vi "Write_Results_file.vi"(0 "Experiment start time":dbl, 1 "Experiment End time":dbl, 3 "Setup filename":string) -> ()   [LabVIEW 2010]
uses:
  Controls/Post_Process.ctl
  Globals/Meas_global.vi
  Globals/Trav_pos_global.vi
  Globals/Dynamic_call_global.ph.vi
panel:
  out "x-y":u32
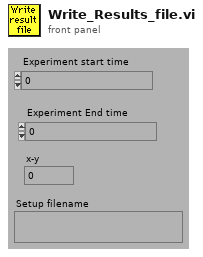
[diagram p1: front panel]
types:
  T1 = typedef "Post_Process.ctl" = enum16{"Take New Data", "Post Process Raw Data File"}
  T2 = cluster{"Name":string, "X":dbl, "Y":dbl, "Z":dbl}[]
  T3 = enum16{"Save no data", "Save data in new files", "Save data in existing files"}
  T4 = typedef "Velocity_cluster.ctl" = cluster{"Name":string, "U":dbl, "u^2":dbl, "u^3/(u^2)^(1.5)":dbl, "u^4/(u^2)^2 -3":dbl, "% u'/U":dbl, "Mean % Err":dbl, "u^4":dbl}
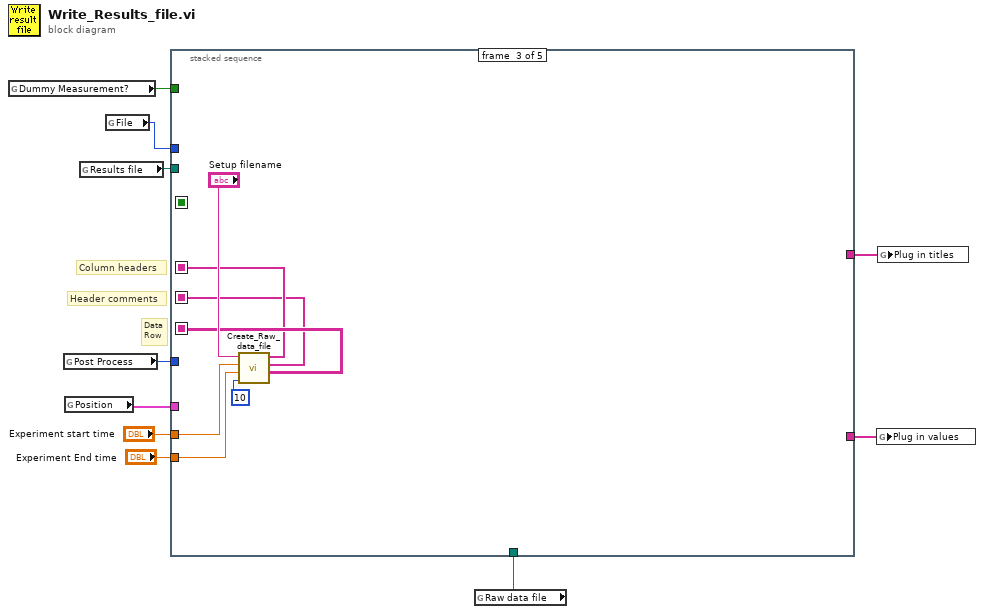
[diagram p0: block diagram]
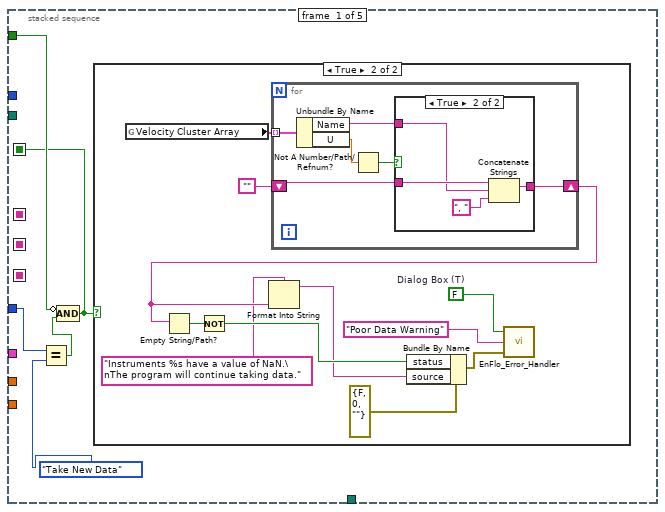
[diagram p2: hidden frame]
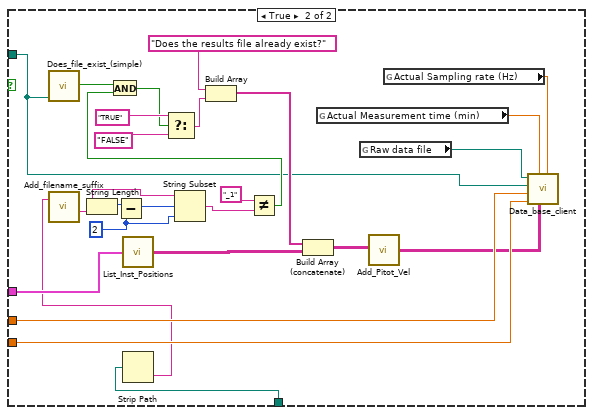
[diagram p6: hidden frame]
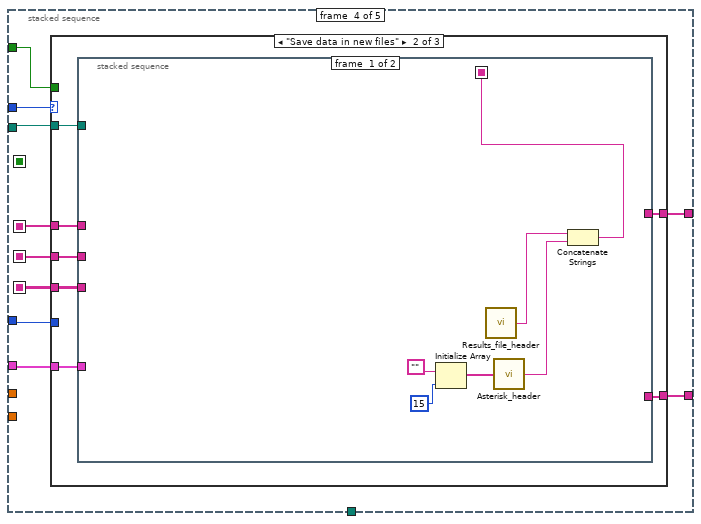
[diagram p7: hidden frame]
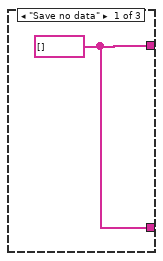
[diagram p8: hidden frame]
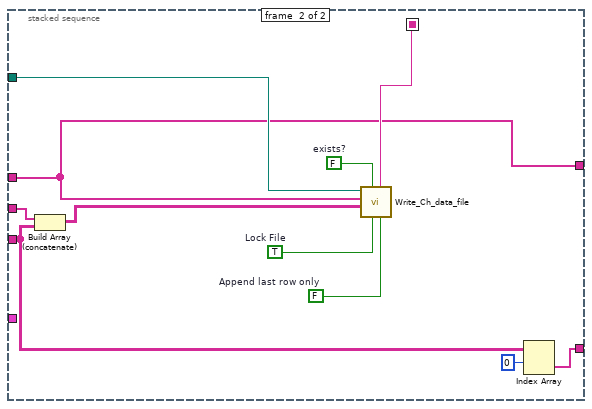
[diagram p9: hidden frame]
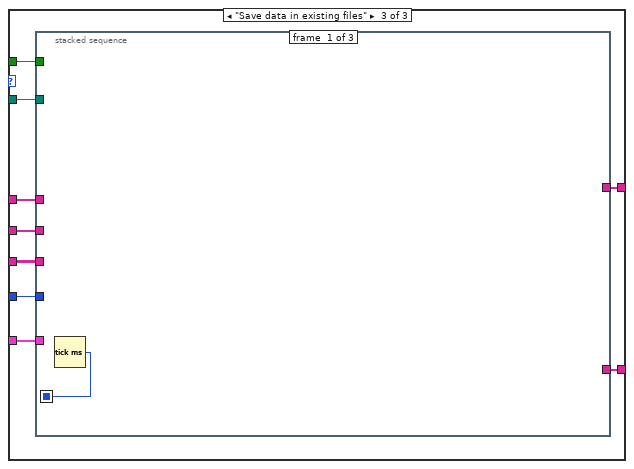
[diagram p10: hidden frame]
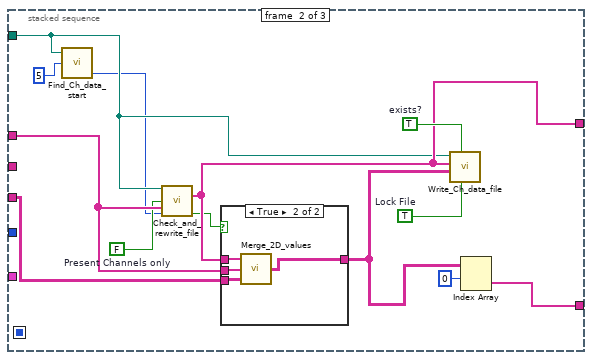
[diagram p11: hidden frame]
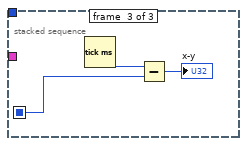
[diagram p13: hidden frame]
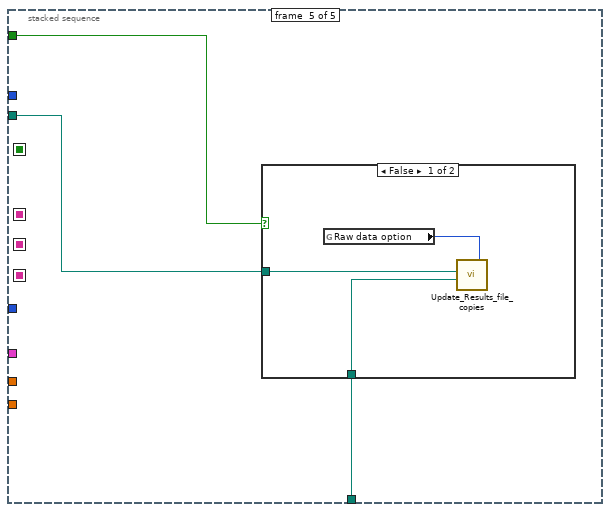
[diagram p14: hidden frame]
diagram:
  # "Data\nRow"
  # "Header comments"
  # "Column headers"
  n1 = global read "Trav_pos_global.vi" "Dummy Measurement?"() -> (w1:bool)
  n2 = global read "Meas_global.vi" "Post Process"() -> (w5:T1)
  n3 = global read "Meas_global.vi" "Position"() -> (w9:T2)
  n4 = global read "Meas_global.vi" "Results file"() -> (w2:path)
  n5 = global read "Meas_global.vi" "File"() -> (w10:T3)
  n6 = global read "Meas_global.vi" "Raw data file"() -> (w8:path)
  n7 = stacked-sequence {
    seq-local: [_ _ w71 _ _] -> [_ _ _ w85 _]
    seq-local: [_ _ w72 _ _] -> [_ _ _ w84 _]
    seq-local: [_ _ w70 _ _] -> [_ _ _ w83 _]
    seq-local: [w11 _ _ _ _] -> [_ w39 _ _ _]
    tunnel: w10 -> [_ _ _ w86 _]
    tunnel: w9 -> [_ w43 _ w82 _]
    tunnel: w8 -> [_ w38 _ _ w145]
    tunnel: "Experiment start time" -> [_ w42 w76 _ _]
    tunnel: "Experiment End time" -> [_ w41 w75 _ _]
    tunnel: w5 -> [w14 _ _ w81 _]
    tunnel: [_ _ _ w80 _] -> w4
    tunnel: [_ _ _ w79 _] -> w3
    tunnel: w2 -> [_ w40 _ w78 w144]
    tunnel: w1 -> [w12 _ _ w77 w143]
    frame #0 {
      n8 = Equal?(x=w14, y=Post_Process."Take New Data" ("Post Process")) -> (x = y?=w13:bool)
      n9 = Compound Arithmetic op=AND(invert w12, w13) -> (w11:bool)
      n10 = case shown="True" w11 {
        frame False {
        }
        frame True {
          w23 = FALSE  # Dialog Box (T)
          n11 = global read "Meas_global.vi" "Velocity Cluster Array"() -> (w26:T4[])
          n12 = for {
            tunnel: w26 -> [w32] mode=indexing
            shift-right: [w27] -> w18
            shift-left: "" -> [w29]
            n13 = Unbundle By Name(w32) -> ("Name"=w28:string, "U"=w31:dbl)
            n14 = Not A Number/Path/Refnum?(number/path/refnum=w31) -> (NaN/Path/Refnum?=w30:bool)
            n15 = case shown="True" w30 {
              tunnel: w29 -> [w33 w37]
              tunnel: w28 -> [_ w36]
              tunnel: [w33 w34] -> w27
              frame False {
              }
              frame True {
                n16 = Concatenate Strings(w37, w36, ", " ("Substring")) -> (w34:string)
              }
            }
          }
          n17 = Empty String/Path?(string/path=w18) -> (empty?=w20:bool)
          n18 = Not(x=w20) -> (.not. x?=w19:bool)
          n19 = Format Into String(format string="Instruments %s have a value of NaN.\nThe program will continue taking data." ("Format String"), w18) -> (resulting string=w16:string)  [unwired: 2 in, 1 out]
          n20 = Bundle By Name(cluster=errorcluster {"status"=FALSE, "code"=0, "source"=""} ("error in (no error)"), "status"=w19, "source"=w16) -> (w21:errorcluster)
          n21 = call "EnFlo_Error_Handler.vi"("error in (no error)"=w21, "Error Type"="Poor Data Warning", "Dialog Box (T)"=w23) -> ()  [unwired: 3 out]
        }
      }
    }
    frame #1 {
      n22 = case shown="False" w39 {
        tunnel: w43 -> [_ w69]
        tunnel: w42 -> [_ w66]
        tunnel: w41 -> [_ w65]
        tunnel: w40 -> [_ w45]
        tunnel: w38 -> [_ w56]
        frame False {
        }
        frame True {
          w51 = 2 ("y")
          n23 = call "Does_file_exist_(simple).vi"("Pathname"=w45) -> ("exists?"=w48:bool)
          n24 = call "List_Inst_Positions.vi"("Position"=w69) -> ("Position Info"=w60:string[][])
          n25 = Strip Path(path=w56) -> (name=w55:string)  [unwired: 1 out]
          n26 = call "Add_filename_suffix.vi"("Filename"=w55) -> ("Base name"=w54:string)  [unwired: 1 in, 3 out]
          n27 = String Length(string=w54) -> (length=w53:i32)
          n28 = Subtract(x=w53, y=w51) -> (x-y=w52:i32)
          n29 = String Subset(string=w54, offset (0)=w52, length (rest)=w51) -> (substring=w50:string)
          n30 = Not Equal?(x="_1", y=w50) -> (x != y?=w47:bool)
          n31 = And(x=w48, y=w47) -> (x .and. y?=w46:bool)
          n32 = Select(t="TRUE", s=w46, f="FALSE") -> (s? t:f=w63:string)
          n33 = Build Array("Does the results file already exist?", w63) -> (w59:string[])
          n34 = Build Array (concatenate)(w59, w60) -> (w58:string[][])
          n35 = global read "Meas_global.vi" "Actual Measurement time (min)"() -> (w68:dbl)
          n36 = global read "Meas_global.vi" "Raw data file"() -> (w44:path)
          n37 = call "Add_Pitot_Vel.vi"("Channels from Client In"=w58) -> ("Channels from Client Out"=w57:string[][])
          n38 = global read "Meas_global.vi" "Actual Sampling rate (Hz)"() -> (w67:dbl)
          n39 = call "Data_base_client.vi"("Average Sampling freq"=w67, "Channels from Client"=w57, "Average Meas Time (min)"=w68, "End time"=w65, "Start time"=w66, "Results File Pathname"=w45, "Raw Data Pathname"=w44) -> ()  [unwired: 4 out]
        }
      }
    }
    frame #2 {
      n40 = call "Create_Raw_data_file.vi"("No of averages"=10, "End time"=w75, "Start time"=w76, "Setup filename"="Setup filename") -> ("Values"=w72:string[][], "Header Comments"=w70:string[], "Column headers"=w71:string[])  [unwired: 1 out]
    }
    frame #3 {
      n41 = case shown="\"Save data in new files\"" w86 {
        tunnel: w85 -> [_ w94 w120]
        tunnel: w84 -> [_ w93 w119]
        tunnel: w83 -> [_ w92 w118]
        tunnel: w78 -> [_ w91 w117]
        tunnel: w82 -> [_ w90 w116]
        tunnel: w81 -> [_ _ w115]
        tunnel: [w87 w88 w114] -> w80
        tunnel: [w87 w89 w113] -> w79
        tunnel: w77 -> [_ _ w112]
        frame "Save no data" {
          w87 = string[] [] ("Merged Channels")
        }
        frame "Save data in new files" {
          n42 = stacked-sequence {
            seq-local: [w95 _] -> [_ w108]
            tunnel: w94 -> [_ w104]
            tunnel: w93 -> [_ w102]
            tunnel: w92 -> [_ w110]
            tunnel: w91 -> [_ w106]
            tunnel: w90 -> [_ _]
            tunnel: [_ w104] -> w89
            tunnel: [_ w101] -> w88
            frame #0 {
              n43 = Initialize Array("", 15) -> (w99:string[])
              n44 = call "Results_file_header.vi"() -> ("Header"=w100:string)
              n45 = call "Asterisk_header.vi"("Channel names"=w99) -> ("Header string"=w96:string)
              n46 = Concatenate Strings(w100, w96) -> (w95:string)
            }
            frame #1 {
              w105 = TRUE  # Lock File
              w107 = FALSE  # Append last row only
              w111 = FALSE  # exists?
              n47 = Build Array (concatenate)(w110, w102) -> (w109:string[][])
              n48 = call "Write_Ch_data_file.vi"("Append last row only"=w107, "Header string"=w108, "Lock File"=w105, "exists?"=w111, "Channel Values"=w109, "Channel names"=w104, "Filename"=w106) -> ()  [unwired: 1 in, 4 out]
              n49 = Index Array(array=w102, index (row)=0) -> (element=w101:string[])  [unwired: 1 in]
            }
          }
        }
        frame "Save data in existing files" {
          n50 = stacked-sequence {
            seq-local: [w121 _ _] -> [_ _ w141]
            tunnel: w120 -> [_ w132 _]
            tunnel: w119 -> [_ w133 _]
            tunnel: w118 -> [_ _ _]
            tunnel: w117 -> [_ w128 _]
            tunnel: w116 -> [_ _ _]
            tunnel: w115 -> [_ _ _]
            tunnel: [_ w122 _] -> w114
            tunnel: [_ w130 _] -> w113
            tunnel: w112 -> [_ _ _]
            frame #0 {
              n51 = Tick Count (ms)() -> (millisecond timer value=w121:u32)
            }
            frame #1 {
              w129 = FALSE  # Present Channels only
              w131 = TRUE  # Lock File
              w134 = TRUE  # exists?
              n52 = call "Find_Ch_data_start.vi"("Approx No Of Columns"=5, "Filename"=w128) -> ("Start of read offset output"=w126:i32)  [unwired: 1 in, 2 out]
              n53 = call "Check_and_rewrite_file.vi"("Filename"=w128, "Present Channels only"=w129, "Present Channels"=w132, "Start of read offset (chars.: 0)"=w126) -> ("Merged Channels"=w130:string[], "Merged?"=w125:bool)  [unwired: 10 out]
              n54 = case shown="True" w125 {
                tunnel: w133 -> [w135 w137]
                tunnel: w132 -> [_ w138]
                tunnel: [w135 w136] -> w123
                tunnel: w130 -> [_ w139]
                frame False {
                }
                frame True {
                  n55 = call "Merge_2D_values.vi"("Values In"=w137, "Present Channels"=w138, "Desired Channels"=w139) -> ("Values Out"=w136:string[][])
                }
              }
              n56 = call "Write_Ch_data_file.vi"("Lock File"=w131, "exists?"=w134, "Channel Values"=w123, "Channel names"=w130, "Filename"=w128) -> ()  [unwired: 3 in, 4 out]
              n57 = Index Array(array=w123, index (row)=0) -> (element=w122:string[])  [unwired: 1 in]
            }
            frame #2 {
              n58 = Tick Count (ms)() -> (millisecond timer value=w142:u32)
              n59 = Subtract(x=w142, y=w141) -> (x-y=→"x-y":u32)
            }
          }
        }
      }
    }
    frame #4 {
      n60 = case shown="False" w143 {
        tunnel: w145 -> [w148 _]
        tunnel: w144 -> [w146 _]
        frame False {
          n61 = global read "Meas_global.vi" "Raw data option"() -> (w147:enum16{"Save raw data", "Raw data not saved"})
          n62 = call "Update_Results_file_copies.vi"("Raw data option"=w147, "Raw data file"=w148, "Results file"=w146) -> ()  [unwired: 4 out]
        }
        frame True {
        }
      }
    }
  }
  n63 = global write "Dynamic_call_global.ph.vi" "Plug in values"(w4) -> ()
  n64 = global write "Dynamic_call_global.ph.vi" "Plug in titles"(w3) -> ()
